vi "Random Competition.vi"() -> ()   [LabVIEW 2024]
uses:
  <vilib>/numeric/Random Number (Range) DBL.vi
panel:
  out "History":cluster{"y":dbl, "y":dbl, dbl[][]}(graph)
  out "Tie":bool
  out "Winner B":bool
  out "Winner A":bool
  out "Points B":dbl
  out "Points A":dbl
  out "Random number B":dbl
  out "Random number A":dbl
  in  "Number of iterations":i32
  # "Guidance\n1. Click on the numeric control \"Number of iterations\" and set its value as the number of iterations you want the program to run.\n2. Run the application.\n3. Embedded random number generators will generate floating-point numbers between -0.5 and 0.5 for A and B. Indicators show the current random number of A and B, the current score of A and B, and the competition result. The history of the competition is shown in a graph."
  # "Input"
  # "Current iteration"
  # "Competition result"
  # "White line: A\nRed line: B"
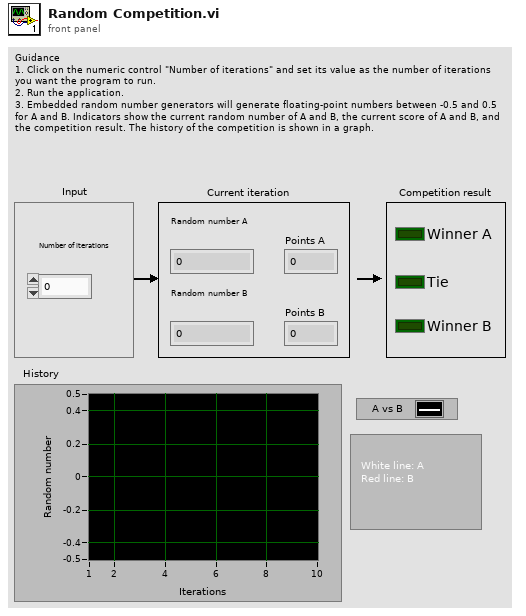
[diagram p1: front panel]
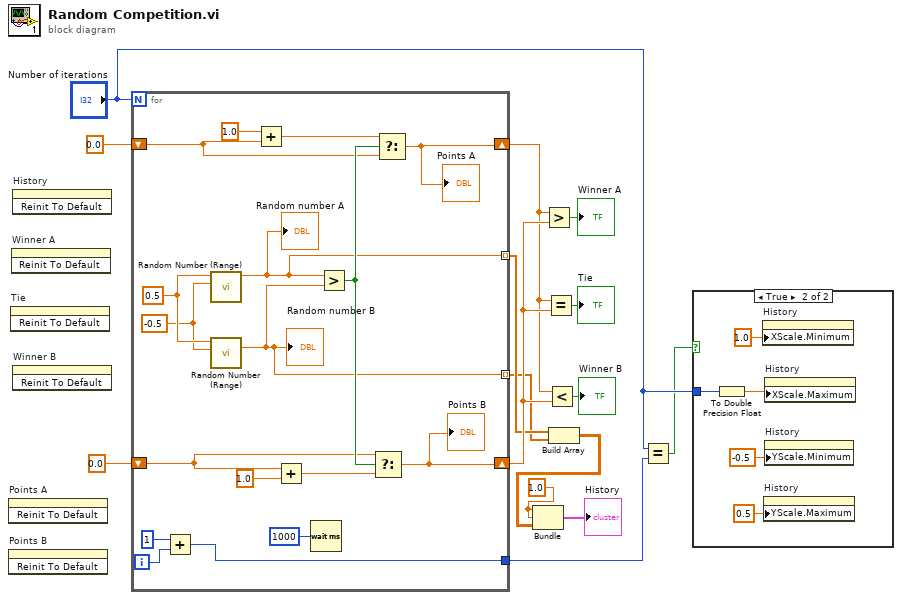
[diagram p0: block diagram]
diagram:
  w8 = 1.0 ("y")
  n1 = invoke on="Points A" class="DigNum (strict)" method="Reinit To Default"() -> ()  [unwired: 3 in, 3 out]
  n2 = invoke on="Points B" class="DigNum (strict)" method="Reinit To Default"() -> ()  [unwired: 3 in, 3 out]
  n3 = invoke on="Tie" class="Bool (strict)" method="Reinit To Default"() -> ()  [unwired: 3 in, 3 out]
  n4 = invoke on="Winner A" class="Bool (strict)" method="Reinit To Default"() -> ()  [unwired: 3 in, 3 out]
  n5 = invoke on="History" class="WFGraph (strict)" method="Reinit To Default"() -> ()  [unwired: 3 in, 3 out]
  n6 = invoke on="Winner B" class="Bool (strict)" method="Reinit To Default"() -> ()  [unwired: 3 in, 3 out]
  n7 = for {
    N: "Number of iterations" -> [_]
    shift-right: [w22] -> w10
    shift-left: 0.0 -> [w27]
    shift-right: [w21] -> w11
    shift-left: 0.0 -> [w24]
    tunnel: [w18] -> w5
    tunnel: [w17] -> w3 mode=indexing
    tunnel: [w16] -> w2 mode=indexing
    i -> [w20]
    w32 = 0.5
    w31 = -0.5
    n8 = Add(x=1, y=w20) -> (x+y=w18:i32)
    n9 = call-poly <vilib>:"Random Number (Range).vi"("lower bound (0)"=w31, "upper bound (100)"=w32) -> ("number"=w17:dbl)  [unwired: 9 in]
    "Random number A" <- w17
    n10 = call-poly <vilib>:"Random Number (Range).vi"("lower bound (0)"=w31, "upper bound (100)"=w32) -> ("number"=w16:dbl)  [unwired: 9 in]
    "Random number B" <- w16
    n11 = Add(x=1.0, y=w27) -> (x+y=w29:dbl)
    n12 = Add(x=w24, y=1.0) -> (x+y=w26:dbl)
    n13 = Wait (ms)(milliseconds to wait=u32 1000) -> ()  [unwired: 1 out]
    n14 = Greater?(x=w17, y=w16) -> (0:w30:bool)
    n15 = Select(t=w24, s=w30, f=w26) -> (s? t:f=w21:dbl)
    "Points B" <- w21
    n16 = Select(t=w29, s=w30, f=w27) -> (s? t:f=w22:dbl)
    "Points A" <- w22
  }
  n17 = Greater?(x=w10, y=w11) -> (0:→"Winner A":bool)
  n18 = Equal?(x=w10, y=w11) -> (x = y?=→"Tie":bool)
  n19 = Less?(x=w10, y=w11) -> (x < y?=→"Winner B":bool)
  n20 = Build Array(w3, w2) -> (w1:dbl[][])
  n21 = Bundle("y"=w8, "y"=w8, w1) -> (→"History":cluster{"y":dbl, "y":dbl, dbl[][]})  [unwired: 1 in]
  n22 = Equal?(x="Number of iterations", y=w5) -> (x = y?=w4:bool)
  n23 = case shown="True" w4 {
    tunnel: "Number of iterations" -> [_ w35]
    frame False {
    }
    frame True {
      n24 = To Double Precision Float(number=w35) -> (double precision float=w36:dbl)
      n25 = property on="History" class="WFGraph (strict)"("XScale.Minimum"=1.0 ("X Scale.Range:Minimum")) -> ()  [unwired: 2 in, 2 out]
      n26 = property on="History" class="WFGraph (strict)"("YScale.Maximum"=0.5 ("Y Scale.Range:Maximum")) -> ()  [unwired: 2 in, 2 out]
      n27 = property on="History" class="WFGraph (strict)"("XScale.Maximum"=w36) -> ()  [unwired: 2 in, 2 out]
      n28 = property on="History" class="WFGraph (strict)"("YScale.Minimum"=-0.5 ("Y Scale.Range:Minimum")) -> ()  [unwired: 2 in, 2 out]
    }
  }
